vi "Read Contents.vi"(8 "error in (no error)":errorcluster, 11 "Element Array":refnum<class "Element Array.lvclass">) -> (0 "error out":errorcluster, 2 "Contents":refnum<class "Data Item.lvclass">[](array[class]), 3 "Element Array Out":refnum<class "Element Array.lvclass">)   [LabVIEW 2020, in "VILab.lvlib" / "Element Array.lvclass"]
uses:
  Element Array.lvclass
  Data Item/Data Item.lvclass
  Element Array.lvclass/Element Array.ctl
  Attribute/Attribute.lvclass
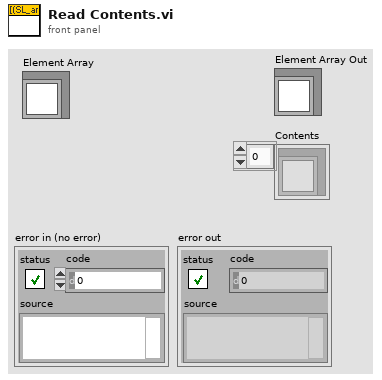
[diagram p1: front panel]
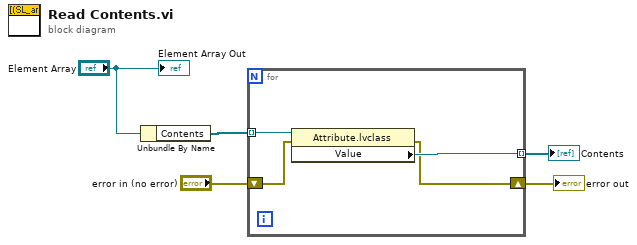
[diagram p0: block diagram]
diagram:
  n1 = Unbundle By Name("Element Array") -> ("Contents"=w4:refnum<class "Attribute.lvclass">[])
  n2 = for {
    tunnel: w4 -> [w9] mode=indexing
    shift-right: [w6] -> w1
    shift-left: "error in (no error)" -> [w8]
    tunnel: [w7] -> w2 mode=indexing
    n3 = property class="Attribute.lvclass"(reference=w9, error in=w8) -> (error out=w6:errorcluster, "Value"=w7:refnum<class "Data Item.lvclass">)  [unwired: 1 out]
  }
  "error out" <- w1
  "Contents" <- w2
  "Element Array Out" <- "Element Array"
